vi "GetRuleTag.vi"(8 "error in (no error)":errorcluster, 11 "HorizontalRule in":refnum<class "HorizontalRule.lvclass">) -> (0 "error out":errorcluster, 2 "RuleTag":string, 3 "HorizontalRule out":refnum<class "HorizontalRule.lvclass">)   [LabVIEW 2021, in "Markdown.lvlib" / "HorizontalRule.lvclass"]
uses:
  HorizontalRule.lvclass
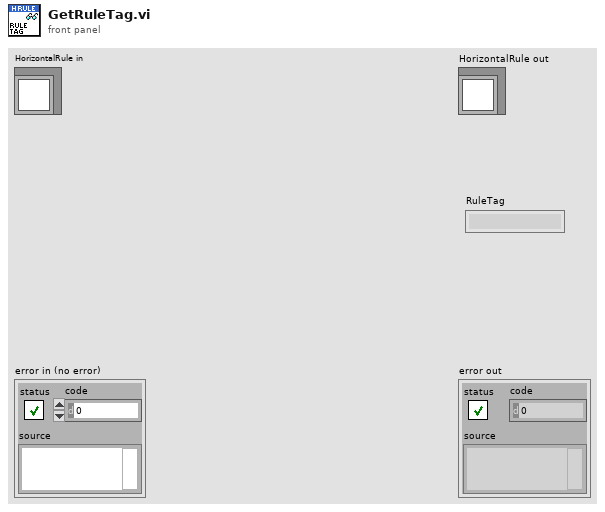
[diagram p1: front panel]
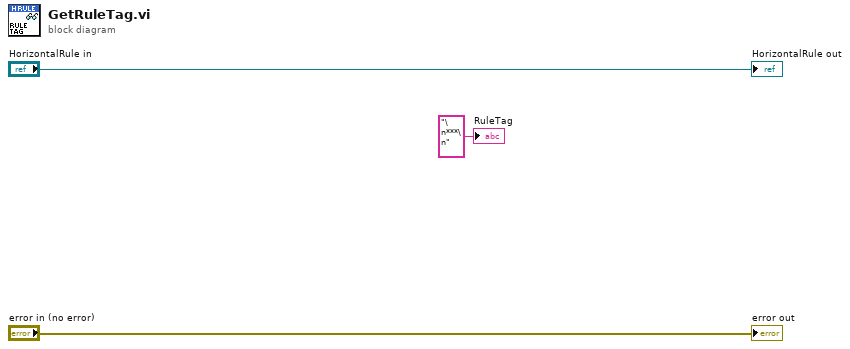
[diagram p0: block diagram]
diagram:
  "error out" <- "error in (no error)"
  "HorizontalRule out" <- "HorizontalRule in"
  "RuleTag" <- "\n***\n" ("RuleTag")
